vi "Autonomous.vi"() -> ()   [LabVIEW 2015]
doc: "This VI starts when autonomous period begins, and will automatically be terminated when it ends. You can carry out timed or sensor driven operations directly to I/O or to subsystems without needing to return to the caller."
uses:
  <vilib>/Rock Robotics/Network Tables/NT Read String.vi
  <vilib>/Utility/file.llb/Read Delimited Spreadsheet (DBL).vi
panel:
  out "Current Row":dbl[](array[numeric])
  out "all rows":dbl[][](array[numeric])
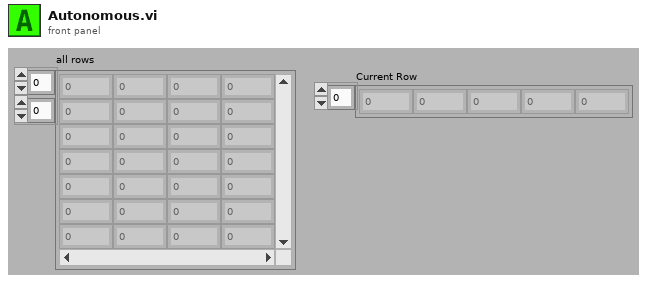
[diagram p1: front panel]
types:
  T1 = typedef "Command Status Info.ctl" = cluster{"Name":string, "Status":T2, "notifier out":T3}
  T2 = typedef "Completion Status.ctl" = enum16{"Successful", "Aborted", "Incomplete"}
  T3 = typedef "Completion Notifier.ctl" = refnum<notifier>
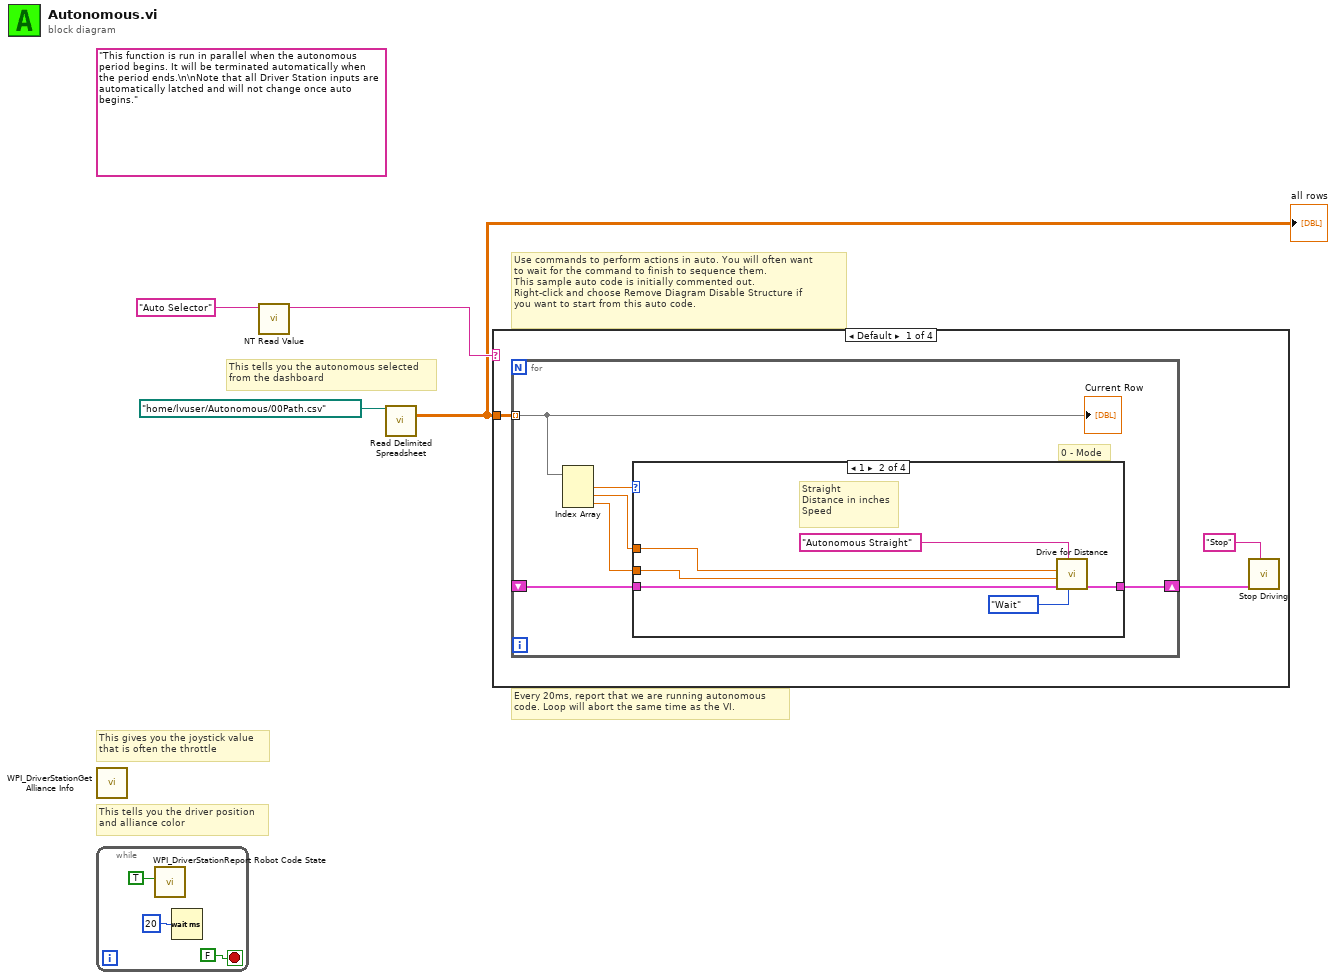
[diagram p0: block diagram]
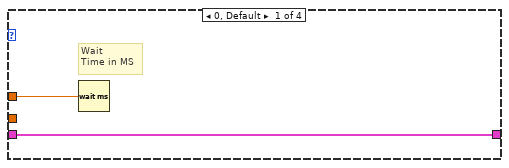
[diagram p2: hidden frame]
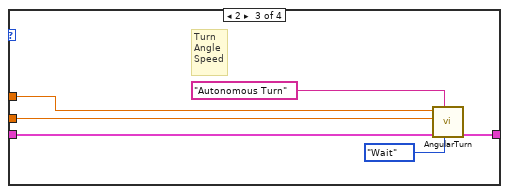
[diagram p3: hidden frame]
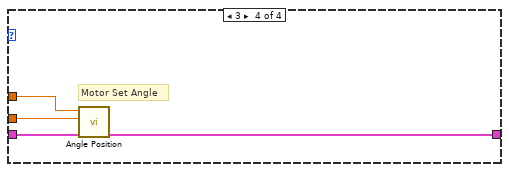
[diagram p4: hidden frame]
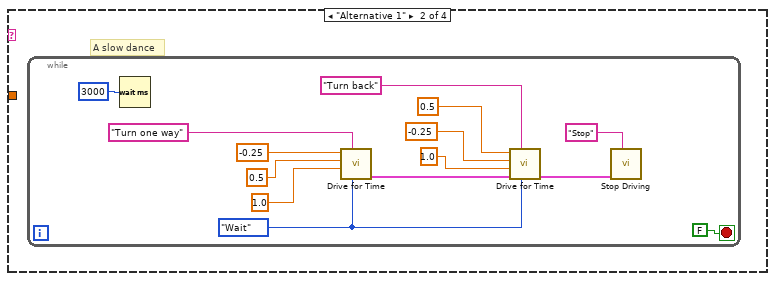
[diagram p5: hidden frame]
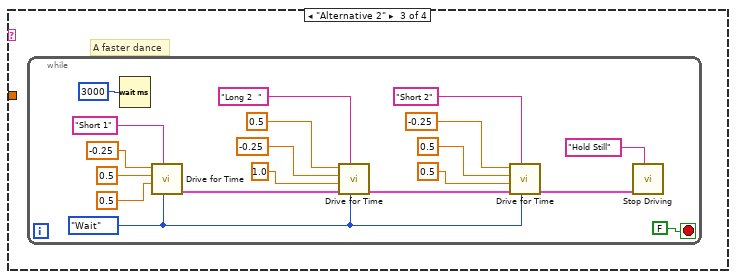
[diagram p6: hidden frame]
diagram:
  (unwired) "This function is run in parallel when the autonomous period begins. It will be terminated automatically when the period ends.\n\nNote that all Driver Station inputs are automatically latched and will not change once auto begins."
  # "This tells you the autonomous selected\nfrom the dashboard"
  # "Every 20ms, report that we are running autonomous\ncode. Loop will abort the same time as the VI."
  # "This gives you the joystick value\nthat is often the throttle"
  # "Use commands to perform actions in auto. You will often want\nto wait for the command to finish to sequence them.\nThis sample auto code is initially commented out. \nRight-click and choose Remove Diagram Disable Structure if\nyou want to start from this auto code."
  # "This tells you the driver position\nand alliance color"
  n1 = call <vilib>:"WPI_DriverStationGet Alliance Info.vi"() -> ()  [unwired: 12 out]
  n2 = while {
    stop <- FALSE stop-if-true
    n3 = call <vilib>:"WPI_DriverStationReport Robot Code State.vi"("Autonomous"=TRUE) -> ()  [unwired: 10 in, 1 out]
    n4 = Wait (ms)(milliseconds to wait=u32 20) -> ()  [unwired: 1 out]
  }
  n5 = call-poly <vilib>:"NT Read Value.vi"("Name"="Auto Selector") -> ("String"=w3:string)  [unwired: 9 in, 1 out]
  n6 = call-poly <vilib>:"Read Delimited Spreadsheet.vi"("file path (dialog if empty)"=path "/home/lvuser/Autonomous/00Path.csv" ("configuration file path")) -> ("all rows"=w1:dbl[][])  [unwired: 9 in, 5 out]
  "all rows" <- w1
  n7 = case shown="Default" w3 {
    tunnel: w1 -> [w10 _ _ _]
    frame Default {
      n8 = for {
        tunnel: w10 -> [w16] mode=indexing
        shift-right: [w11] -> w9
        shift-left: _ -> [w12]
        # "0 - Mode"
        n9 = Index Array(array=w16) -> (element #1=w15:dbl, element #2=w14:dbl, element #3=w13:dbl)  [unwired: 3 in]
        n10 = case shown="1" w15 {
          tunnel: w14 -> [w17 w20 w30 w34]
          tunnel: w13 -> [_ w21 w29 w33]
          tunnel: w12 -> [w18 w24 w27 w32]
          tunnel: [w18 w23 w26 w31] -> w11
          frame 0, Default {
            # "Wait\nTime in MS"
            n11 = Wait (ms)(milliseconds to wait=w17) -> ()  [unwired: 1 out]
          }
          frame 1 {
            # "Straight\nDistance in inches\nSpeed"
            n12 = call "Drive for Distance.vi"("Synchronization"=enum16{"Start", "Wait"}."Wait", "Description"="Autonomous Straight", "Command Info In"=w24, "Speed"=w21, "Distance (in)"=w20) -> ("Command Info Out"=w23:T1)  [unwired: 5 in, 1 out]
          }
          frame 2 {
            # "Turn\nAngle\nSpeed"
            n13 = call "AngularTurn.vi"("Synchronization"=enum16{"Start", "Wait"}."Wait", "Description"="Autonomous Turn", "Command Info In"=w27, "Speed"=w29, "Angle To Turn"=w30) -> ("Command Info Out"=w26:T1)  [unwired: 5 in, 1 out]
          }
          frame 3 {
            # "Motor Set Angle"
            n14 = call "Angle Position.vi"("Command Info In"=w32, "Angle"=w33, "Motor ID"=w34) -> ("Command Info"=w31:T1)  [unwired: 8 in]
          }
        }
        "Current Row" <- w16
      }
      n15 = call "Stop Driving.vi"("Description"="Stop", "Command Info In"=w9) -> ()  [unwired: 9 in, 1 out]
    }
    frame "Alternative 1" {
      # "A slow dance"
      n16 = while {
        stop <- FALSE stop-if-true
        w39 = enum16{"Start", "Wait"}."Wait" ("Synchronication")
        n17 = Wait (ms)(milliseconds to wait=u32 3000 ("millisecond timer value")) -> ()  [unwired: 1 out]
        n18 = call "Drive for Time.vi"("Synchronization"=w39, "Description"="Turn one way", "Seconds"=1.0 ("Delay (s)"), "Right Speed"=0.5 ("X axis value"), "Left Speed"=-0.25 ("X axis value")) -> ("Command Info Out"=w48:T1)  [unwired: 5 in, 1 out]
        n19 = call "Drive for Time.vi"("Synchronization"=w39, "Description"="Turn back", "Command Info In"=w48, "Seconds"=1.0 ("Delay (s)"), "Right Speed"=-0.25 ("X axis value"), "Left Speed"=0.5 ("X axis value")) -> ("Command Info Out"=w38:T1)  [unwired: 4 in, 1 out]
        n20 = call "Stop Driving.vi"("Description"="Stop", "Command Info In"=w38) -> ()  [unwired: 9 in, 1 out]
      }
    }
    frame "Alternative 2" {
      # "A faster dance"
      n21 = while {
        stop <- FALSE stop-if-true
        w49 = enum16{"Start", "Wait"}."Wait" ("Synchronication")
        n22 = Wait (ms)(milliseconds to wait=u32 3000 ("millisecond timer value")) -> ()  [unwired: 1 out]
        n23 = call "Drive for Time.vi"("Synchronization"=w49, "Description"="Short 1", "Seconds"=0.5 ("Delay (s)"), "Right Speed"=0.5 ("X axis value"), "Left Speed"=-0.25 ("X axis value")) -> ("Command Info Out"=w67:T1)  [unwired: 5 in, 1 out]
        n24 = call "Drive for Time.vi"("Synchronization"=w49, "Description"="Long 2  ", "Command Info In"=w67, "Seconds"=1.0 ("Delay (s)"), "Right Speed"=-0.25 ("X axis value"), "Left Speed"=0.5 ("X axis value")) -> ("Command Info Out"=w51:T1)  [unwired: 4 in, 1 out]
        n25 = call "Drive for Time.vi"("Synchronization"=w49, "Description"="Short 2", "Command Info In"=w51, "Seconds"=0.5 ("Delay (s)"), "Right Speed"=0.5 ("X axis value"), "Left Speed"=-0.25 ("X axis value")) -> ("Command Info Out"=w50:T1)  [unwired: 4 in, 1 out]
        n26 = call "Stop Driving.vi"("Description"="Hold Still", "Command Info In"=w50) -> ()  [unwired: 9 in, 1 out]
      }
    }
    frame "Your Turn" {
    }
  }
